vi "High Resolution Timing.vi"(2 "relative seconds (NaN)":dbl=nan, 3 "Error In":errorcluster) -> (10 "relative seconds":dbl, 16 "elapsed (relative) seconds":dbl, 17 "Error Out":errorcluster)   [LabVIEW 2019]
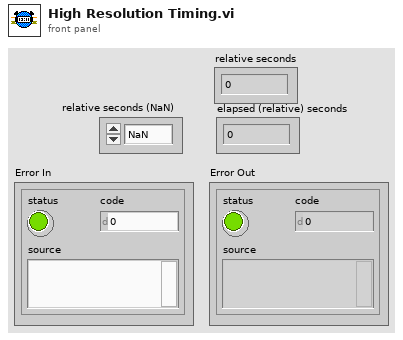
[diagram p1: front panel]
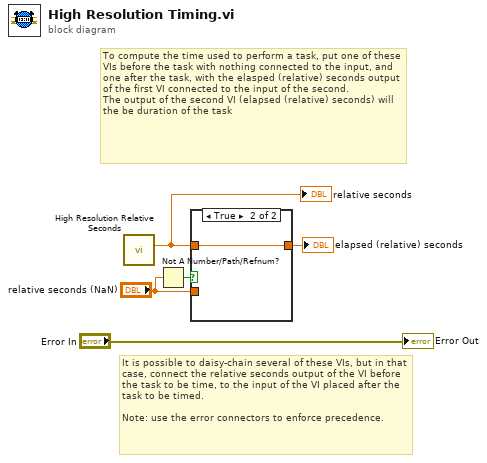
[diagram p0: block diagram]
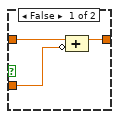
[diagram p2: hidden frame]
diagram:
  # "It is possible to daisy-chain several of these VIs, but in that case, connect the relative seconds output of the VI before the task to be time, to the input of the VI placed after the task to be timed.\n\nNote: use the error connectors to enforce precedence."
  # "To compute the time used to perform a task, put one of these VIs before the task with nothing connected to the input, and one after the task, with the elasped (relative) seconds output of the first VI connected to the input of the second.\nThe output of the second VI (elapsed (relative) seconds) will the be duration of the task"
  n1 = call <vilib>:"High Resolution Relative Seconds.vi"() -> ("relative seconds"=w1:dbl)
  "relative seconds" <- w1
  n2 = Not A Number/Path/Refnum?(number/path/refnum="relative seconds (NaN)") -> (NaN/Path/Refnum?=w3:bool)
  n3 = case shown="True" w3 {
    tunnel: "relative seconds (NaN)" -> [w8 _]
    tunnel: [w7 w9] -> w5
    tunnel: w1 -> [w6 w9]
    frame False {
      n4 = Compound Arithmetic op=ADD(w6, invert w8) -> (w7:dbl)
    }
    frame True {
    }
  }
  "elapsed (relative) seconds" <- w5
  "Error Out" <- "Error In"
